vi "2_2.vi"() -> ()   [LabVIEW 2021]
panel:
  out "x*y":i32
  out "Vertical (depth)":i32
  out "Horizontal":i32
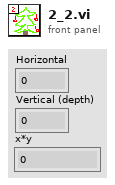
[diagram p1: front panel]
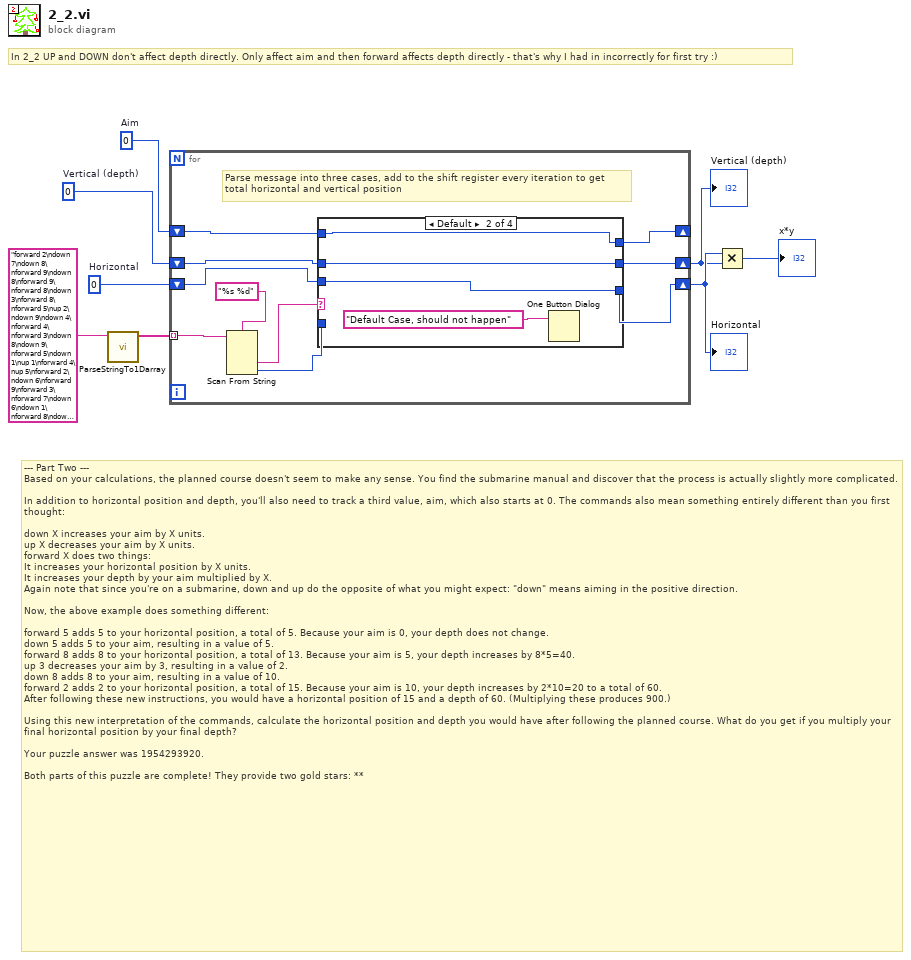
[diagram p0: block diagram]
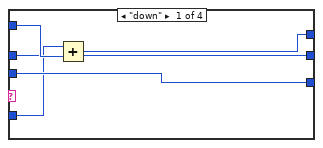
[diagram p2: hidden frame]
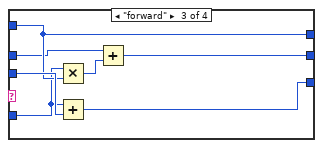
[diagram p3: hidden frame]
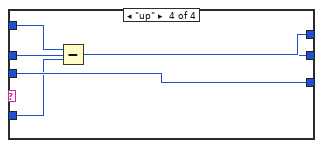
[diagram p4: hidden frame]
diagram:
  w1 = 0  # Aim
  w7 = 0  # Vertical (depth)
  w8 = 0  # Horizontal
  # "--- Part Two ---\nBased on your calculations, the planned course doesn't seem to make any sense. You find the submarine manual and discover that the process is actually slightly more complicated.\n\nIn addition to horizontal position and depth, you'll also need to track a third value, aim, which also starts at 0. The commands also mean something entirely different than you first thought:\n\ndown X increases your aim by X units.\nup X decreases your aim by X units.\nforward X does two things:\nIt increases your horizontal position by X units.\nIt increases your depth by your aim multiplied by X.\nAgain note that since you're on a submarine, down and up do the opposite of what you might expect: \"down\" means aiming in the positive direction.\n\nNow, the above example does something different:\n\nforward 5 adds 5 to your horizontal position, a total of 5. Because your aim is 0, your depth does not change.\ndown 5 adds 5 to your aim, resulting in a value of 5.\nforward 8 adds 8 to your horizontal position, a total of 13. Because your aim is 5, your depth increases by 8*5=40.\nup 3 decreases your aim by 3, resulting in a value of 2.\ndown 8 adds 8 to your aim, resulting in a value of 10.\nforward 2 adds 2 to your horizontal position, a total of 15. Because your aim is 10, your depth increases by 2*10=20 to a total of 60.\nAfter following these new instructions, you would have a horizontal position of 15 and a depth of 60. (Multiplying these produces 900.)\n\nUsing this new interpretation of the commands, calculate the horizontal position and depth you would have after following the planned course. What do you get if you multiply your final horizontal position by your final depth?\n\nYour puzzle answer was 1954293920.\n\nBoth parts of this puzzle are complete! They provide two gold stars: **"
  # "In 2_2 UP and DOWN don't affect depth directly. Only affect aim and then forward affects depth directly - that's why I had in incorrectly for first try :)"
  n1 = call "ParseStringTo1Darray.vi"("Copied Input From Advent Of Code Website"="forward 2\ndown 7\ndown 8\nforward 9\ndown 8\nforward 9\nforward 8\ndown 3\nforward 8\nforward 5\nup 2\ndown 9\ndown 4\nforward 4\nforward 3\ndown 8\ndown 9\nforward 5\ndown 1\nup 1\nforward 4\nup 5\nforward 2\ndown 6\nforward 9\nforward 3\nforward 7\ndown 6\ndown 1\nforward 8\ndown 3\nforward 1\nup 6\ndown 1\ndown 2\nforward 9\ndown 7\ndown 1\ndown 7\ndown 7\nup 5\ndown 8\nforward 6\nup 8\nup 2\nforward 6\nup 1\ndown 9\nforward 8\nforward 4\nup 3\nforward 7\ndown 2\ndown 8\nforward 5\ndown 9\nup 4\nforward 7\nforward 5\ndown 5\ndown 5\nforward 3\nforward 2\ndown 2\nup 4\nup 7\ndown 8\nup 8\nforward 1\nup 4\nforward 4\ndown 2\nforward 5\nforward 7\ndown 4\nforward 8\ndown 2\nforward 5\nforward 9\nforward 6\nforward 5\ndown 5\nforward 4\nforward 3\ndown 7\ndown 8\nforward 9\nforward 7\ndown 3\ndown 6\nforward 4\ndown 7\nup 9\ndown 8\nup 7\nup 3\nforward 6\nforward 9\ndown 2\ndown 3\ndown 1\ndown 3\nforward 8\nforward 3\nforward 9\ndown 5\nup 1\nup 2\ndown 9\nup 9\ndown 5\ndown 9\nforward 1\ndown 3\ndown 5\ndown 1\nforward 7\ndown 6\nforward 7\nforward 4\nup 2\nup 1\nforward 9\ndown 2\ndown 6\ndown 5\ndown 6\nforward 8\ndown 5\nforward 1\nforward 2\ndown 7\ndown 5\ndown 7\nup 9\ndown 9\nup 4\ndown 7\nup 8\ndown 9\nforward 3\ndown 6\ndown 2\nforward 9\ndown 4\nup 7\nforward 3\ndown 5\nforward 8\nforward 9\ndown 2\nup 5\nforward 2\nforward 9\nup 5\ndown 2\nforward 8\nforward 6\ndown 7\ndown 3\nforward 4\nforward 3\nforward 9\nup 4\nup 4\nforward 7\nup 3\nforward 6\ndown 7\nup 8\nforward 2\nup 1\ndown 6\nforward 4\nup 6\nup 6\nup 3\nforward 4\nforward 2\nforward 5\nforward 8\ndown 9\ndown 4\ndown 3\ndown 1\ndown 6\ndown 4\ndown 5\ndown 7\ndown 5\nup 4\nforward 3\ndown 4\ndown 7\ndown 7\ndown 2\nforward 2\nforward 9\nup 6\ndown 3\nup 9\nforward 8\ndown 9\nup 2\nup 2\nup 2\nup 1\ndown 6\nforward 9\nforward 2\nforward 2\nforward 2\nforward 5\nup 3\ndown 7\ndown 6\ndown 8\nup 3\nup 9\ndown 3\nforward 1\nforward 7\ndown 7\ndown 1\nforward 3\ndown 7\ndown 9\ndown 7\ndown 3\nup 2\ndown 6\nup 6\ndown 1\nup 2\nforward 7\nup 2\ndown 7\nup 2\ndown 9\ndown 3\nforward 6\ndown 5\ndown 1\nforward 5\ndown 2\ndown 6\ndown 1\ndown 3\ndown 3\ndown 5\nforward 2\nforward 4\nforward 8\nforward 6\nforward 4\nforward 9\nup 8\ndown 5\nforward 1\ndown 1\nforward 1\nforward 6\nup 1\ndown 6\ndown 3\nforward 9\nforward 5\nforward 4\nup 3\nup 7\ndown 2\nup 4\nup 2\ndown 1\nforward 6\nforward 9\nforward 4\nforward 2\ndown 8\nforward 4\nforward 3\nup 5\ndown 4\nforward 3\ndown 8\ndown 5\ndown 5\nforward 1\nforward 6\nforward 4\nforward 5\nforward 9\nforward 5\ndown 4\nforward 3\nforward 8\ndown 8\ndown 1\nup 4\ndown 4\nup 7\nforward 2\nforward 6\ndown 3\ndown 5\ndown 5\ndown 8\nup 3\ndown 2\nforward 4\nforward 2\nforward 4\nforward 9\nup 2\ndown 7\nup 7\ndown 2\nforward 4\nup 7\nforward 4\ndown 2\nforward 7\nup 2\ndown 3\nforward 5\ndown 7\ndown 2\nup 2\nup 1\nup 7\nup 9\ndown 3\nforward 1\nforward 3\ndown 2\ndown 3\nforward 6\ndown 7\nforward 9\ndown 9\nforward 3\nforward 2\ndown 1\nup 9\ndown 4\nforward 4\nup 4\nforward 7\nup 3\ndown 4\ndown 9\ndown 3\nforward 7\ndown 6\ndown 7\ndown 6\nup 5\nforward 3\nforward 9\nup 2\nup 4\nup 9\ndown 2\nforward 5\nup 1\ndown 7\ndown 5\nup 2\nforward 8\ndown 8\nup 3\nforward 4\ndown 9\nforward 6\ndown 9\ndown 5\nforward 6\ndown 8\nup 6\ndown 3\nforward 6\nforward 3\ndown 3\ndown 5\ndown 7\ndown 1\ndown 5\ndown 7\ndown 5\nforward 3\ndown 2\nforward 4\nup 4\nup 1\nup 7\nforward 1\nforward 5\ndown 4\ndown 8\ndown 3\nforward 4\ndown 3\nup 7\ndown 6\nforward 9\nup 8\nforward 2\nforward 5\ndown 6\nup 4\nforward 8\nforward 5\ndown 6\nforward 2\ndown 7\nforward 3\nforward 1\nforward 6\ndown 9\nup 6\ndown 4\ndown 2\nup 8\nforward 4\ndown 8\nforward 8\nup 9\nforward 7\ndown 6\nup 9\ndown 4\nup 6\ndown 4\ndown 3\nup 7\nup 4\nforward 5\nup 9\ndown 9\nup 6\ndown 3\nforward 8\ndown 9\nforward 7\nup 3\nup 9\nforward 8\ndown 3\nforward 3\nforward 5\ndown 6\nforward 3\ndown 4\nup 6\nforward 3\nforward 7\ndown 1\ndown 6\ndown 4\nforward 6\nup 6\ndown 5\ndown 6\ndown 4\nup 2\ndown 7\ndown 9\ndown 2\ndown 6\nforward 3\nforward 4\ndown 5\nup 5\ndown 5\nforward 3\nforward 6\ndown 4\ndown 7\nup 2\nforward 7\ndown 7\nup 6\nup 3\nforward 9\nforward 8\nup 6\nforward 2\ndown 2\nforward 8\nforward 4\nup 6\nforward 6\ndown 8\nup 3\nup 5\nforward 6\nup 8\ndown 1\ndown 4\nup 9\nforward 6\nup 5\ndown 6\ndown 8\ndown 9\nforward 5\nup 3\ndown 7\nforward 3\nforward 6\ndown 3\ndown 1\ndown 9\nup 9\ndown 4\ndown 7\nforward 2\nforward 4\ndown 7\nforward 7\nup 5\ndown 9\nup 7\ndown 4\nforward 6\ndown 5\nforward 4\nup 8\ndown 4\ndown 7\nforward 3\ndown 6\ndown 1\nforward 3\ndown 4\nup 6\nup 5\nup 7\nforward 5\ndown 4\nforward 7\nup 1\ndown 4\nforward 4\ndown 2\ndown 6\nforward 1\nup 3\nup 8\nforward 6\nforward 6\ndown 5\nforward 7\ndown 6\ndown 8\nforward 6\ndown 6\nforward 3\nforward 5\ndown 9\ndown 5\nup 4\ndown 5\ndown 1\nforward 1\nforward 5\ndown 2\nforward 5\nforward 2\nforward 5\nup 3\nforward 5\nup 8\nforward 9\nforward 3\ndown 2\nup 2\nforward 7\ndown 5\nup 1\ndown 3\ndown 7\nup 2\nforward 8\nforward 6\nforward 1\nforward 6\nforward 6\ndown 5\nforward 4\ndown 5\nforward 9\nforward 7\ndown 7\ndown 7\ndown 9\nforward 4\ndown 4\nforward 3\ndown 6\nforward 5\ndown 9\nforward 6\nup 7\ndown 3\nup 4\nup 4\ndown 1\ndown 2\nup 5\nforward 6\nforward 2\ndown 7\nup 6\nup 3\ndown 8\nforward 1\ndown 3\nup 9\ndown 2\nforward 6\nforward 1\nforward 4\nup 1\ndown 8\ndown 2\ndown 9\ndown 5\nforward 3\ndown 1\ndown 6\ndown 5\ndown 3\nforward 1\nforward 9\nup 2\ndown 3\ndown 3\ndown 9\ndown 7\nforward 6\nforward 8\nforward 4\nup 7\ndown 2\nforward 3\nforward 1\nup 4\nforward 8\nup 9\nforward 8\nforward 2\ndown 5\nforward 2\ndown 6\ndown 6\ndown 4\nforward 8\ndown 6\nforward 2\nforward 8\ndown 7\ndown 6\nforward 2\ndown 1\ndown 8\nforward 2\nforward 9\nup 6\nforward 6\ndown 3\ndown 2\nup 5\nup 6\ndown 6\nup 7\nforward 5\nforward 7\ndown 1\nforward 7\nforward 9\ndown 3\nforward 4\nforward 5\ndown 1\nup 3\nforward 2\nup 5\nforward 2\nforward 1\ndown 5\ndown 4\ndown 8\nup 8\nforward 3\ndown 3\nforward 4\ndown 6\nup 8\ndown 5\nup 2\ndown 1\nup 3\nforward 8\nup 6\nforward 9\nup 9\ndown 5\nforward 2\nforward 9\nup 6\nforward 1\ndown 2\nforward 4\nforward 4\nforward 1\nforward 5\nforward 1\nforward 4\ndown 5\ndown 1\ndown 2\ndown 2\nforward 7\ndown 7\ndown 7\ndown 4\ndown 7\ndown 4\ndown 3\nup 7\nup 1\nforward 2\nforward 3\ndown 4\ndown 5\nforward 9\nup 7\nforward 6\ndown 1\nforward 6\nforward 6\nforward 8\ndown 3\nforward 2\ndown 6\nforward 9\nup 6\nup 6\nforward 7\ndown 5\ndown 6\nup 3\ndown 5\nup 4\nforward 3\ndown 7\nforward 9\nup 1\ndown 1\nup 6\ndown 3\nup 2\ndown 5\nforward 3\nforward 6\ndown 9\ndown 4\nforward 7\ndown 1\nup 1\nforward 3\nforward 5\nup 7\ndown 3\nup 9\nup 9\ndown 4\nup 4\nforward 8\nup 9\ndown 8\nforward 6\nforward 4\nforward 9\nforward 8\ndown 2\nforward 3\nforward 2\ndown 3\nup 1\nforward 6\ndown 3\ndown 7\ndown 3\ndown 5\ndown 9\nup 9\nforward 8\nforward 6\ndown 8\nforward 3\ndown 4\ndown 2\ndown 9\nforward 4\nforward 2\nup 4\nforward 1\nup 8\nup 1\ndown 4\nup 2\ndown 1\nup 7\ndown 2\ndown 4\nup 4\nforward 2\ndown 3\nforward 2\nforward 3\ndown 5\nforward 9\nforward 7\ndown 1\nup 3\ndown 3\nforward 3\ndown 6\nforward 5\nup 3\nup 3\nup 1\nforward 7\nforward 1\nforward 2\nforward 2\ndown 4\nup 7\nforward 1\nforward 1\nforward 6\ndown 8\nup 8\ndown 8\ndown 4\ndown 6\nforward 8\nforward 4\nforward 5\ndown 2\ndown 3\nforward 7\ndown 6\nforward 4\nforward 1\nup 7\nup 5\nup 2\nforward 1\nforward 8\nforward 2\nup 9\nforward 4\nforward 5\ndown 2\nforward 5\nforward 7\ndown 3\nforward 1\ndown 3\nup 5\nup 2\nup 2\nup 2\nforward 4\nforward 4\nforward 8\nforward 2\ndown 3\nup 7\ndown 4\ndown 2\ndown 7\nforward 2\ndown 2\nforward 7\nup 9\nup 7\nforward 7\nforward 7\ndown 3\ndown 4\nup 4\ndown 2\ndown 8\nforward 4\ndown 1\nup 6\nforward 4\ndown 2\nup 8\ndown 1\ndown 8\ndown 6\nup 9\nforward 4\nup 1\ndown 2\ndown 9\ndown 7\ndown 4\ndown 8\ndown 8\nup 1\ndown 5\nup 5\ndown 7\nup 7\nforward 5\ndown 3\nforward 7\nup 5\ndown 3\nforward 9\nup 5\ndown 7\nforward 8\nforward 8\ndown 2\nforward 7\nforward 8\ndown 4\nup 7\ndown 2\nup 7\nforward 5\ndown 1\ndown 3\nforward 9\nup 4\nforward 6\nforward 4\ndown 5\ndown 7\nforward 2\nforward 4\ndown 2\nforward 1\ndown 5\nup 2\ndown 8\ndown 1\ndown 4\ndown 8\ndown 6\nforward 9\nforward 2\nforward 6\nforward 4\ndown 1\nforward 8\nup 4\nforward 6\ndown 4\nforward 4\nforward 3\nforward 6\nforward 9\nforward 8\ndown 1\nforward 5\ndown 8\nforward 7\nup 1\ndown 3\nup 6\nforward 5\nforward 8\nforward 8\nforward 5\nforward 5\nforward 1\nup 9\nforward 7\nup 3\ndown 2\ndown 4\nforward 6\nup 2\nforward 5\nup 8\nforward 8\nforward 2\nforward 6\nforward 3\nup 4\nforward 3\nforward 6" ("String")) -> ("Formatted 1D String Array"=w5:string[])  [unwired: 10 in]
  n2 = for {
    shift-right: [w12] -> w3
    shift-left: w7 -> [w13]
    shift-right: [w14] -> w4
    shift-left: w8 -> [w15]
    tunnel: w5 -> [w18] mode=indexing
    shift-right: [w9] -> _
    shift-left: w1 -> [w10]
    # "Parse message into three cases, add to the shift register every iteration to get \ntotal horizontal and vertical position"
    n3 = Scan From String(format string="%s %d", input string=w18) -> (output 1=w16:string, output 2=w11:i32)  [unwired: 4 in, 3 out]
    n4 = case shown="Default" w16 {
      tunnel: w15 -> [w23 w27 w34 w39]
      tunnel: [w23 w27 w33 w39] -> w14
      tunnel: w13 -> [w19 w26 w29 w35]
      tunnel: [w19 w26 w28 w35] -> w12
      tunnel: w11 -> [w20 _ w31 w37]
      tunnel: w10 -> [w22 w24 w32 w38]
      tunnel: [w21 w24 w32 w36] -> w9
      frame "down" {
        n5 = Add(x=w20, y=w22) -> (x+y=w21:i32)
      }
      frame Default {
        n6 = One Button Dialog(message="Default Case, should not happen") -> ()  [unwired: 1 in, 1 out]
      }
      frame "forward" {
        n7 = Multiply(x=w31, y=w32) -> (x*y=w30:i32)
        n8 = Add(x=w31, y=w34) -> (x+y=w33:i32)
        n9 = Add(x=w29, y=w30) -> (x+y=w28:i32)
      }
      frame "up" {
        n10 = Subtract(x=w38, y=w37) -> (x-y=w36:i32)
      }
    }
  }
  "Horizontal" <- w4
  "Vertical (depth)" <- w3
  n11 = Multiply(x=w4, y=w3) -> (x*y=→"x*y":i32)
